vi "Communicator - Passive1.v.vi"() -> ()   [LabVIEW 2019]
panel:
  out "MC_Receive":T1 {"MirrorCoverControlScheme"."Time" format="%<%Y-%m-%d %H:%M:%S>T"; "MirrorCoverControllerConfig"."Time" format="%<%Y-%m-%d %H:%M:%S>T"; "MirrorCoverMotor-All"."MirrorCoverMotor-00"."Time" format="%<%Y-%m-%d %H:%M:%S>T"; "MirrorCoverMotor-All"."MirrorCoverMotor-01"."Time" format="%<%Y-%m-%d %H:%M:%S>T"; "MirrorCoverMotor-All"."MirrorCoverMotor-02"."Time" format="%<%Y-%m-%d %H:%M:%S>T"; "MirrorCoverMotor-All"."MirrorCoverMotor-03"."Time" format="%<%Y-%m-%d %H:%M:%S>T"; "MirrorCoverMotor-All"."MirrorCoverMotor-04"."Time" format="%<%Y-%m-%d %H:%M:%S>T"; "MirrorCoverMotor-All"."MirrorCoverMotor-05"."Time" format="%<%Y-%m-%d %H:%M:%S>T"; "MirrorCoverMotor-All"."MirrorCoverMotor-06"."Time" format="%<%Y-%m-%d %H:%M:%S>T"; "MirrorCoverMotor-All"."MirrorCoverMotor-07"."Time" format="%<%Y-%m-%d %H:%M:%S>T"}
  out "MC_Send 2":T1 {"MirrorCoverControlScheme"."Time" format="%<%Y-%m-%d %H:%M:%S>T"; "MirrorCoverControllerConfig"."Time" format="%<%Y-%m-%d %H:%M:%S>T"; "MirrorCoverMotor-All"."MirrorCoverMotor-00"."Time" format="%<%Y-%m-%d %H:%M:%S>T"; "MirrorCoverMotor-All"."MirrorCoverMotor-01"."Time" format="%<%Y-%m-%d %H:%M:%S>T"; "MirrorCoverMotor-All"."MirrorCoverMotor-02"."Time" format="%<%Y-%m-%d %H:%M:%S>T"; "MirrorCoverMotor-All"."MirrorCoverMotor-03"."Time" format="%<%Y-%m-%d %H:%M:%S>T"; "MirrorCoverMotor-All"."MirrorCoverMotor-04"."Time" format="%<%Y-%m-%d %H:%M:%S>T"; "MirrorCoverMotor-All"."MirrorCoverMotor-05"."Time" format="%<%Y-%m-%d %H:%M:%S>T"; "MirrorCoverMotor-All"."MirrorCoverMotor-06"."Time" format="%<%Y-%m-%d %H:%M:%S>T"; "MirrorCoverMotor-All"."MirrorCoverMotor-07"."Time" format="%<%Y-%m-%d %H:%M:%S>T"}
  in  "MC_Send":T1 {"MirrorCoverControlScheme"."Time" format="%<%Y-%m-%d %H:%M:%S>T"; "MirrorCoverControllerConfig"."Time" format="%<%Y-%m-%d %H:%M:%S>T"; "MirrorCoverMotor-All"."MirrorCoverMotor-00"."Time" format="%<%Y-%m-%d %H:%M:%S>T"; "MirrorCoverMotor-All"."MirrorCoverMotor-01"."Time" format="%<%Y-%m-%d %H:%M:%S>T"; "MirrorCoverMotor-All"."MirrorCoverMotor-02"."Time" format="%<%Y-%m-%d %H:%M:%S>T"; "MirrorCoverMotor-All"."MirrorCoverMotor-03"."Time" format="%<%Y-%m-%d %H:%M:%S>T"; "MirrorCoverMotor-All"."MirrorCoverMotor-04"."Time" format="%<%Y-%m-%d %H:%M:%S>T"; "MirrorCoverMotor-All"."MirrorCoverMotor-05"."Time" format="%<%Y-%m-%d %H:%M:%S>T"; "MirrorCoverMotor-All"."MirrorCoverMotor-06"."Time" format="%<%Y-%m-%d %H:%M:%S>T"; "MirrorCoverMotor-All"."MirrorCoverMotor-07"."Time" format="%<%Y-%m-%d %H:%M:%S>T"}
  in  "Port":u16=6342
  in  "stop":bool
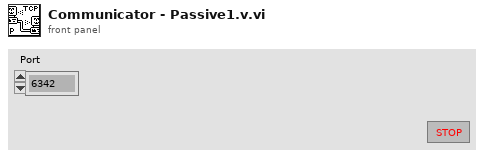
[diagram p1: front panel]
types:
  T1 = cluster{"MirrorCoverControlScheme":cluster{"Cold Start":bool, "Configuration":bool, "Start":bool, "Pointing/Tracking":bool, "Standby":bool, "Stop":bool, "Shutdown":bool, "Start Calibration":bool, "Start Maintenance":bool, "Status":i16, "Time ":timestamp}, "MirrorCoverControllerConfig":cluster{"ID":dbl, "K_P Config":dbl, "K_I Config":dbl, "K_D Config":dbl, "Status":i16, "Time ":timestamp}, "MirrorCoverMotor-All":cluster{"MirrorCoverMotor-00":cluster{"ID":i32, "Enable":bool, "Direction":bool, "Brake":bool, "Built-In Encoder":u64, "Motor Voltage FB":bool, "Motor Current FB":u64, "Brake Voltage FB":bool, "Brake Current FB":u64, "Up Limit Switch":bool, "Down Limit Switch":bool, "Up Limit Config":u64, "Down Limit Config":u64, "Motor Current Limit Config":u64, "Brake Current Limit Config":u64, "Status":i16, "Time ":timestamp}, "MirrorCoverMotor-01":cluster{"ID":i32, "Enable":bool, "Direction":bool, "Brake":bool, "Built-In Encoder":u64, "Motor Voltage FB":bool, "Motor Current FB":u64, "Brake Voltage FB":bool, "Brake Current FB":u64, "Up Limit Switch":bool, "Down Limit Switch":bool, "Up Limit Config":u64, "Down Limit Config":u64, "Motor Current Limit Config":u64, "Brake Current Limit Config":u64, "Status":i16, "Time ":timestamp}, "MirrorCoverMotor-02":cluster{"ID":i32, "Enable":bool, "Direction":bool, "Brake":bool, "Built-In Encoder":u64, "Motor Voltage FB":bool, "Motor Current FB":u64, "Brake Voltage FB":bool, "Brake Current FB":u64, "Up Limit Switch":bool, "Down Limit Switch":bool, "Up Limit Config":u64, "Down Limit Config":u64, "Motor Current Limit Config":u64, "Brake Current Limit Config":u64, "Status":i16, "Time ":timestamp}, "MirrorCoverMotor-03":cluster{"ID":i32, "Enable":bool, "Direction":bool, "Brake":bool, "Built-In Encoder":u64, "Motor Voltage FB":bool, "Motor Current FB":u64, "Brake Voltage FB":bool, "Brake Current FB":u64, "Up Limit Switch":bool, "Down Limit Switch":bool, "Up Limit Config":u64, "Down Limit Config":u64, "Motor Current Limit Config":u64, "Brake Current Limit Config":u64, "Status":i16, "Time ":timestamp}, "MirrorCoverMotor-04":cluster{"ID":i32, "Enable":bool, "Direction":bool, "Brake":bool, "Built-In Encoder":u64, "Motor Voltage FB":bool, "Motor Current FB":u64, "Brake Voltage FB":bool, "Brake Current FB":u64, "Up Limit Switch":bool, "Down Limit Switch":bool, "Up Limit Config":u64, "Down Limit Config":u64, "Motor Current Limit Config":u64, "Brake Current Limit Config":u64, "Status":i16, "Time ":timestamp}, "MirrorCoverMotor-05":cluster{"ID":i32, "Enable":bool, "Direction":bool, "Brake":bool, "Built-In Encoder":u64, "Motor Voltage FB":bool, "Motor Current FB":u64, "Brake Voltage FB":bool, "Brake Current FB":u64, "Up Limit Switch":bool, "Down Limit Switch":bool, "Up Limit Config":u64, "Down Limit Config":u64, "Motor Current Limit Config":u64, "Brake Current Limit Config":u64, "Status":i16, "Time ":timestamp}, "MirrorCoverMotor-06":cluster{"ID":i32, "Enable":bool, "Direction":bool, "Brake":bool, "Built-In Encoder":u64, "Motor Voltage FB":bool, "Motor Current FB":u64, "Brake Voltage FB":bool, "Brake Current FB":u64, "Up Limit Switch":bool, "Down Limit Switch":bool, "Up Limit Config":u64, "Down Limit Config":u64, "Motor Current Limit Config":u64, "Brake Current Limit Config":u64, "Status":i16, "Time ":timestamp}, "MirrorCoverMotor-07":cluster{"ID":i32, "Enable":bool, "Direction":bool, "Brake":bool, "Built-In Encoder":u64, "Motor Voltage FB":bool, "Motor Current FB":u64, "Brake Voltage FB":bool, "Brake Current FB":u64, "Up Limit Switch":bool, "Down Limit Switch":bool, "Up Limit Config":u64, "Down Limit Config":u64, "Motor Current Limit Config":u64, "Brake Current Limit Config":u64, "Status":i16, "Time ":timestamp}}}
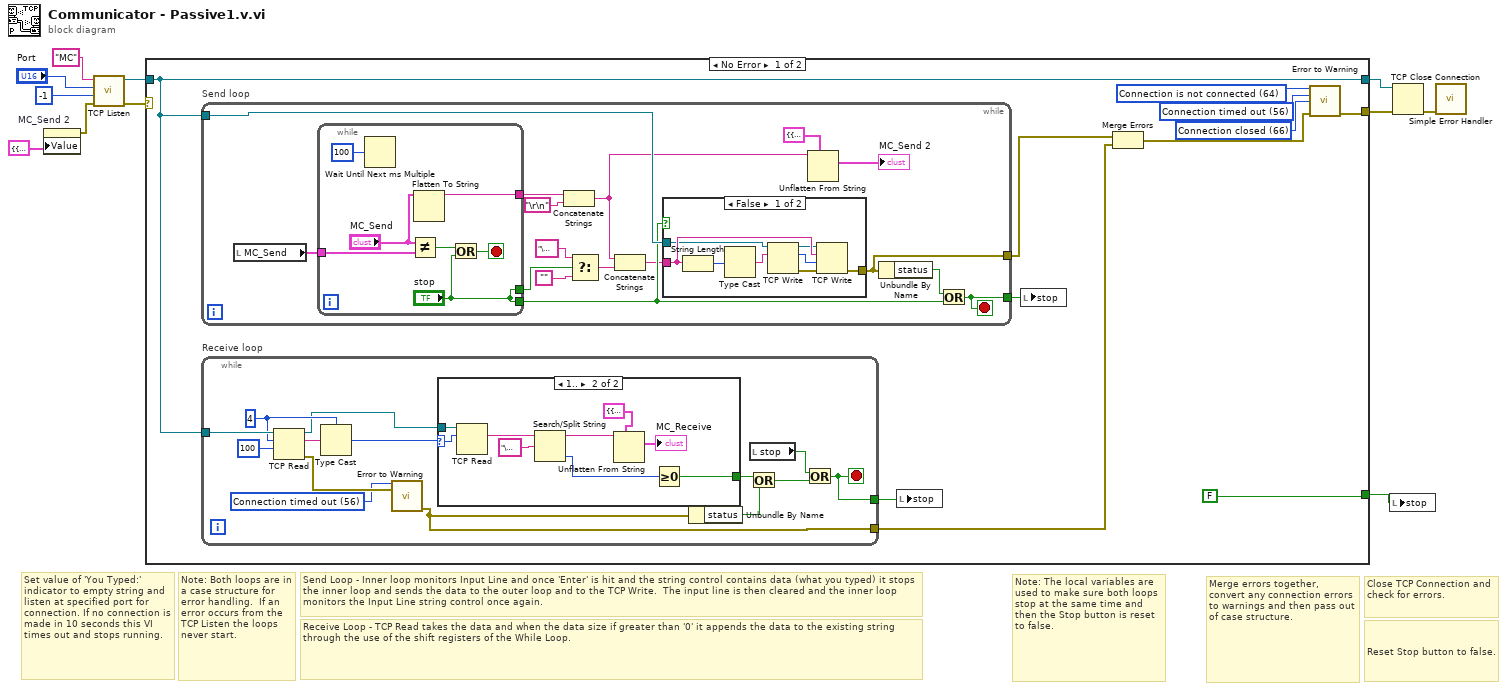
[diagram p0: block diagram]
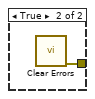
[diagram p2: hidden frame]
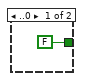
[diagram p3: hidden frame]
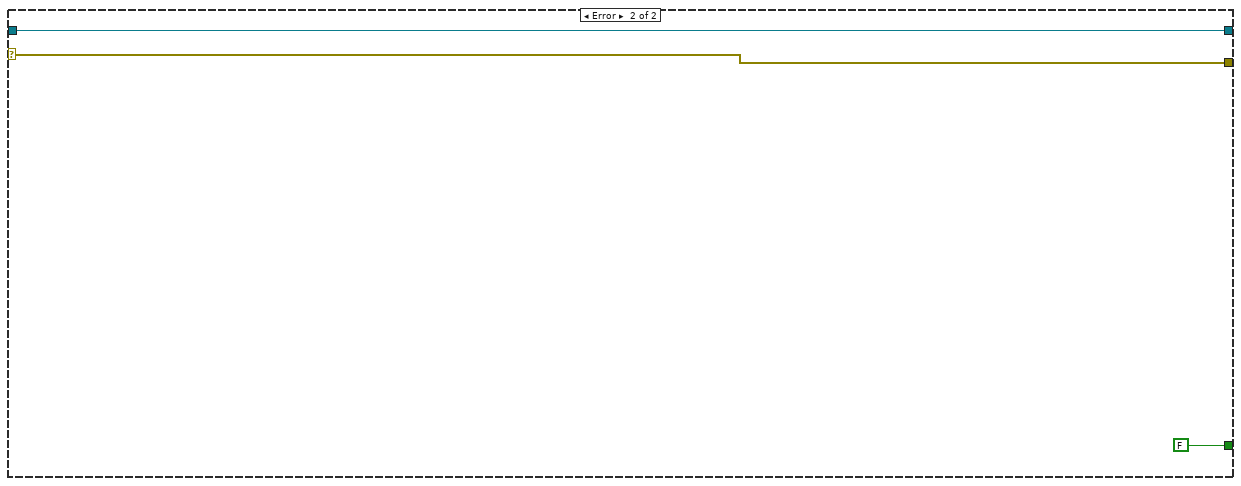
[diagram p4: hidden frame]
diagram:
  # "Reset Stop button to false."
  # "Close TCP Connection and check for errors."
  # "Note: Both loops are in a case structure for error handling.  If an error occurs from the TCP Listen the loops never start."
  # "Merge errors together, convert any connection errors to warnings and then pass out of case structure."
  # "Note: The local variables are used to make sure both loops stop at the same time and then the Stop button is reset to false."
  # "Receive Loop - TCP Read takes the data and when the data size if greater than '0' it appends the data to the existing string through the use of the shift registers of the While Loop."
  # "Send Loop - Inner loop monitors Input Line and once 'Enter' is hit and the string control contains data (what you typed) it stops the inner loop and sends the data to the outer loop and to the TCP Write.  The input line is then cleared and the inner loop monitors the Input Line string control once again."
  # "Set value of 'You Typed:' indicator to empty string and listen at specified port for connection. If no connection is made in 10 seconds this VI times out and stops running."
  n1 = property on="MC_Send 2" class="Clust (strict)"("Value"=T1 {"MirrorCoverControlScheme"={"Cold Start"=FALSE, "Configuration"=FALSE, "Start"=FALSE, "Pointing/Tracking"=FALSE, "Standby"=FALSE, "Stop"=FALSE, "Shutdown"=FALSE, "Start Calibration"=FALSE, "Start Maintenance"=FALSE, "Status"=0, "Time "=timestamp(0 s since 1904-01-01)}, "MirrorCoverControllerConfig"={"ID"=0.0, "K_P Config"=0.0, "K_I Config"=0.0, "K_D Config"=0.0, "Status"=0, "Time "=timestamp(0 s since 1904-01-01)}, "MirrorCoverMotor-All"={"MirrorCoverMotor-00"={"ID"=0, "Enable"=FALSE, "Direction"=FALSE, "Brake"=FALSE, "Built-In Encoder"=0, "Motor Voltage FB"=FALSE, "Motor Current FB"=0, "Brake Voltage FB"=FALSE, "Brake Current FB"=0, "Up Limit Switch"=FALSE, "Down Limit Switch"=FALSE, "Up Limit Config"=0, "Down Limit Config"=0, "Motor Current Limit Config"=0, "Brake Current Limit Config"=0, "Status"=0, "Time "=timestamp(0 s since 1904-01-01)}, "MirrorCoverMotor-01"={"ID"=0, "Enable"=FALSE, "Direction"=FALSE, "Brake"=FALSE, "Built-In Encoder"=0, "Motor Voltage FB"=FALSE, "Motor Current FB"=0, "Brake Voltage FB"=FALSE, "Brake Current FB"=0, "Up Limit Switch"=FALSE, "Down Limit Switch"=FALSE, "Up Limit Config"=0, "Down Limit Config"=0, "Motor Current Limit Config"=0, "Brake Current Limit Config"=0, "Status"=0, "Time "=timestamp(0 s since 1904-01-01)}, "MirrorCoverMotor-02"={"ID"=0, "Enable"=FALSE, "Direction"=FALSE, "Brake"=FALSE, "Built-In Encoder"=0, "Motor Voltage FB"=FALSE, "Motor Current FB"=0, "Brake Voltage FB"=FALSE, "Brake Current FB"=0, "Up Limit Switch"=FALSE, "Down Limit Switch"=FALSE, "Up Limit Config"=0, "Down Limit Config"=0, "Motor Current Limit Config"=0, "Brake Current Limit Config"=0, "Status"=0, "Time "=timestamp(0 s since 1904-01-01)}, "MirrorCoverMotor-03"={"ID"=0, "Enable"=FALSE, "Direction"=FALSE, "Brake"=FALSE, "Built-In Encoder"=0, "Motor Voltage FB"=FALSE, "Motor Current FB"=0, "Brake Voltage FB"=FALSE, "Brake Current FB"=0, "Up Limit Switch"=FALSE, "Down Limit Switch"=FALSE, "Up Limit Config"=0, "Down Limit Config"=0, "Motor Current Limit Config"=0, "Brake Current Limit Config"=0, "Status"=0, "Time "=timestamp(0 s since 1904-01-01)}, "MirrorCoverMotor-04"={"ID"=0, "Enable"=FALSE, "Direction"=FALSE, "Brake"=FALSE, "Built-In Encoder"=0, "Motor Voltage FB"=FALSE, "Motor Current FB"=0, "Brake Voltage FB"=FALSE, "Brake Current FB"=0, "Up Limit Switch"=FALSE, "Down Limit Switch"=FALSE, "Up Limit Config"=0, "Down Limit Config"=0, "Motor Current Limit Config"=0, "Brake Current Limit Config"=0, "Status"=0, "Time "=timestamp(0 s since 1904-01-01)}, "MirrorCoverMotor-05"={"ID"=0, "Enable"=FALSE, "Direction"=FALSE, "Brake"=FALSE, "Built-In Encoder"=0, "Motor Voltage FB"=FALSE, "Motor Current FB"=0, "Brake Voltage FB"=FALSE, "Brake Current FB"=0, "Up Limit Switch"=FALSE, "Down Limit Switch"=FALSE, "Up Limit Config"=0, "Down Limit Config"=0, "Motor Current Limit Config"=0, "Brake Current Limit Config"=0, "Status"=0, "Time "=timestamp(0 s since 1904-01-01)}, "MirrorCoverMotor-06"={"ID"=0, "Enable"=FALSE, "Direction"=FALSE, "Brake"=FALSE, "Built-In Encoder"=0, "Motor Voltage FB"=FALSE, "Motor Current FB"=0, "Brake Voltage FB"=FALSE, "Brake Current FB"=0, "Up Limit Switch"=FALSE, "Down Limit Switch"=FALSE, "Up Limit Config"=0, "Down Limit Config"=0, "Motor Current Limit Config"=0, "Brake Current Limit Config"=0, "Status"=0, "Time "=timestamp(0 s since 1904-01-01)}, "MirrorCoverMotor-07"={"ID"=0, "Enable"=FALSE, "Direction"=FALSE, "Brake"=FALSE, "Built-In Encoder"=0, "Motor Voltage FB"=FALSE, "Motor Current FB"=0, "Brake Voltage FB"=FALSE, "Brake Current FB"=0, "Up Limit Switch"=FALSE, "Down Limit Switch"=FALSE, "Up Limit Config"=0, "Down Limit Config"=0, "Motor Current Limit Config"=0, "Brake Current Limit Config"=0, "Status"=0, "Time "=timestamp(0 s since 1904-01-01)}}} ("MC_Receive")) -> (error out=w6:errorcluster)  [unwired: 2 in, 1 out]
  n2 = call <vilib>:"TCP Listen.vi"("error in (no error)"=w6, "timeout ms (wait forever: -1)"=-1, "port"="Port", "service name"="MC") -> ("error out"=w7:errorcluster, "connection ID"=w8:refnum<k5>)  [unwired: 3 in, 3 out]
  n3 = case shown="No Error" w7 {
    selector: w7 -> [_ w80]
    tunnel: [w17 w80] -> w10
    tunnel: w8 -> [w12 w81]
    tunnel: [w12 w81] -> w11
    tunnel: [FALSE FALSE] -> w3
    frame No Error {
      w14 = 56 items=["No Error", "Argument Error", "Memory Full", "Out of Zone", "End of File", "File Already Open", "Generic File IO Error", "File Not Found", "File Permission Error", "Disk Full", "Duplicate Path", "Too Many Files Open", "Not Enabled", "Resource File Not Found", "Cannot Add Resource", "Resource Not Found", "Image Not Found", "Image Memory Error", "Pen Does Not Exist", "Config Bad Type", "Config Token Not Found", "Config Parse Error", "Config Memory Error", "Bad External Code Format", "Bad External Code Offset", "External Code Not Present", "Null Window", "Destroy Window Mixup", "Null Menu", "Print Aborted", "Bad Print Record", "Print Driver Error", "Windows Error During Print", "Memory Error During Print", "Print Dialog Error", "Generic Print Error", "Invalid Device Refnum", "Device Not Found", "Device Parameter Error", "Device Unit Error", "Can't Open Device", "Device Call Aborted", "Generic Error", "Cancelled By User", "Object ID Too Low", "Object ID Too High", "Object Not In Heap", "Unknown Heap", "Bad DefProc ID", "DefProc Not In Table", "Message Out Of Range", "Null Method", "Unknown Message", "Manager Call Not Supported", "Bad address", "Connection In progress", "Connection timed out", "Connection is already in progress", "Network attribute not supported", "Network error", "Address in use", "System out of memory", "Connection aborted", "Connection refused", "Connection is not connected", "Connection is already connected", "Connection closed", "Initialize error (interapplication manager)", "Bad occurrence", "Wait on unbound occurrence handler", "Occurrence queue overflow", "Bad path", "Semaphore not signaled", "Unrecognized type (interapplication manager)"] ("2nd Error to Convert")
      w18 = 66 items=["No Error", "Argument Error", "Memory Full", "Out of Zone", "End of File", "File Already Open", "Generic File IO Error", "File Not Found", "File Permission Error", "Disk Full", "Duplicate Path", "Too Many Files Open", "Not Enabled", "Resource File Not Found", "Cannot Add Resource", "Resource Not Found", "Image Not Found", "Image Memory Error", "Pen Does Not Exist", "Config Bad Type", "Config Token Not Found", "Config Parse Error", "Config Memory Error", "Bad External Code Format", "Bad External Code Offset", "External Code Not Present", "Null Window", "Destroy Window Mixup", "Null Menu", "Print Aborted", "Bad Print Record", "Print Driver Error", "Windows Error During Print", "Memory Error During Print", "Print Dialog Error", "Generic Print Error", "Invalid Device Refnum", "Device Not Found", "Device Parameter Error", "Device Unit Error", "Can't Open Device", "Device Call Aborted", "Generic Error", "Cancelled By User", "Object ID Too Low", "Object ID Too High", "Object Not In Heap", "Unknown Heap", "Bad DefProc ID", "DefProc Not In Table", "Message Out Of Range", "Null Method", "Unknown Message", "Manager Call Not Supported", "Bad address", "Connection In progress", "Connection timed out", "Connection is already in progress", "Network attribute not supported", "Network error", "Address in use", "System out of memory", "Connection aborted", "Connection refused", "Connection is not connected", "Connection is already connected", "Connection closed", "Initialize error (interapplication manager)", "Bad occurrence", "Wait on unbound occurrence handler", "Occurrence queue overflow", "Bad path", "Semaphore not signaled", "Unrecognized type (interapplication manager)"] ("3rd Error to Convert")
      w19 = 64 items=["No Error", "Argument Error", "Memory Full", "Out of Zone", "End of File", "File Already Open", "Generic File IO Error", "File Not Found", "File Permission Error", "Disk Full", "Duplicate Path", "Too Many Files Open", "Not Enabled", "Resource File Not Found", "Cannot Add Resource", "Resource Not Found", "Image Not Found", "Image Memory Error", "Pen Does Not Exist", "Config Bad Type", "Config Token Not Found", "Config Parse Error", "Config Memory Error", "Bad External Code Format", "Bad External Code Offset", "External Code Not Present", "Null Window", "Destroy Window Mixup", "Null Menu", "Print Aborted", "Bad Print Record", "Print Driver Error", "Windows Error During Print", "Memory Error During Print", "Print Dialog Error", "Generic Print Error", "Invalid Device Refnum", "Device Not Found", "Device Parameter Error", "Device Unit Error", "Can't Open Device", "Device Call Aborted", "Generic Error", "Cancelled By User", "Object ID Too Low", "Object ID Too High", "Object Not In Heap", "Unknown Heap", "Bad DefProc ID", "DefProc Not In Table", "Message Out Of Range", "Null Method", "Unknown Message", "Manager Call Not Supported", "Bad address", "Connection In progress", "Connection timed out", "Connection is already in progress", "Network attribute not supported", "Network error", "Address in use", "System out of memory", "Connection aborted", "Connection refused", "Connection is not connected", "Connection is already connected", "Connection closed", "Initialize error (interapplication manager)", "Bad occurrence", "Wait on unbound occurrence handler", "Occurrence queue overflow", "Bad path", "Semaphore not signaled", "Unrecognized type (interapplication manager)"] ("1st Error to Convert")
      n4 = while "Send loop" {
        tunnel: w12 -> [w37]
        tunnel: [w38] -> w15
        tunnel: [w33] -> w21
        stop <- w38 stop-if-true
        n5 = local read "MC_Send"() -> (w30:T1)
        n6 = while {
          tunnel: ["stop"] -> w35
          tunnel: ["stop"] -> w31
          tunnel: [w39] -> w26
          tunnel: w30 -> [w42]
          stop <- w43 stop-if-true
          n7 = Wait Until Next ms Multiple(millisecond multiple=u32 100) -> ()  [unwired: 1 out]
          n8 = Not Equal?(x="MC_Send", y=w42) -> (x != y?=w44:bool)
          n9 = Flatten To String(anything="MC_Send") -> (data string=w39:string)  [unwired: 3 in, 2 out]
          n10 = Or(x=w44, y="stop") -> (x .or. y?=w43:bool)
        }
        n11 = Concatenate Strings(w26, "\r\n") -> (w25:string)
        n12 = Select(t="\u0004", s=w35, f="") -> (s? t:f=w24:string)
        n13 = Concatenate Strings(w25, w24) -> (w23:string)
        n14 = case shown="False" w31 {
          tunnel: w23 -> [w50 _]
          tunnel: [w53 w54] -> w33
          tunnel: w37 -> [w47 _]
          frame False {
            n15 = String Length(string=w50) -> (length=w49:i32)
            n16 = Type Cast(x=w49) -> (*(type *) &x=w48:string)  [unwired: 1 in]
            n17 = TCP Write(connection ID=w47, data in=w48) -> (connection ID out=w46:refnum<k5>, bytes written=w51:i32, error out=w52:errorcluster)  [unwired: 2 in]
            n18 = TCP Write(connection ID=w46, data in=w50, error in (no error)=w52, 9:w51) -> (error out=w53:errorcluster)  [unwired: 2 out]
          }
          frame True {
            n19 = call <vilib>:"Clear Errors.vi"() -> ("error out"=w54:errorcluster)  [unwired: 6 in, 1 out]
          }
        }
        n20 = Unflatten From String(type=T1 {"MirrorCoverControlScheme"={"Cold Start"=FALSE, "Configuration"=FALSE, "Start"=FALSE, "Pointing/Tracking"=FALSE, "Standby"=FALSE, "Stop"=FALSE, "Shutdown"=FALSE, "Start Calibration"=FALSE, "Start Maintenance"=FALSE, "Status"=0, "Time "=timestamp(0 s since 1904-01-01)}, "MirrorCoverControllerConfig"={"ID"=0.0, "K_P Config"=0.0, "K_I Config"=0.0, "K_D Config"=0.0, "Status"=0, "Time "=timestamp(0 s since 1904-01-01)}, "MirrorCoverMotor-All"={"MirrorCoverMotor-00"={"ID"=0, "Enable"=FALSE, "Direction"=FALSE, "Brake"=FALSE, "Built-In Encoder"=0, "Motor Voltage FB"=FALSE, "Motor Current FB"=0, "Brake Voltage FB"=FALSE, "Brake Current FB"=0, "Up Limit Switch"=FALSE, "Down Limit Switch"=FALSE, "Up Limit Config"=0, "Down Limit Config"=0, "Motor Current Limit Config"=0, "Brake Current Limit Config"=0, "Status"=0, "Time "=timestamp(0 s since 1904-01-01)}, "MirrorCoverMotor-01"={"ID"=0, "Enable"=FALSE, "Direction"=FALSE, "Brake"=FALSE, "Built-In Encoder"=0, "Motor Voltage FB"=FALSE, "Motor Current FB"=0, "Brake Voltage FB"=FALSE, "Brake Current FB"=0, "Up Limit Switch"=FALSE, "Down Limit Switch"=FALSE, "Up Limit Config"=0, "Down Limit Config"=0, "Motor Current Limit Config"=0, "Brake Current Limit Config"=0, "Status"=0, "Time "=timestamp(0 s since 1904-01-01)}, "MirrorCoverMotor-02"={"ID"=0, "Enable"=FALSE, "Direction"=FALSE, "Brake"=FALSE, "Built-In Encoder"=0, "Motor Voltage FB"=FALSE, "Motor Current FB"=0, "Brake Voltage FB"=FALSE, "Brake Current FB"=0, "Up Limit Switch"=FALSE, "Down Limit Switch"=FALSE, "Up Limit Config"=0, "Down Limit Config"=0, "Motor Current Limit Config"=0, "Brake Current Limit Config"=0, "Status"=0, "Time "=timestamp(0 s since 1904-01-01)}, "MirrorCoverMotor-03"={"ID"=0, "Enable"=FALSE, "Direction"=FALSE, "Brake"=FALSE, "Built-In Encoder"=0, "Motor Voltage FB"=FALSE, "Motor Current FB"=0, "Brake Voltage FB"=FALSE, "Brake Current FB"=0, "Up Limit Switch"=FALSE, "Down Limit Switch"=FALSE, "Up Limit Config"=0, "Down Limit Config"=0, "Motor Current Limit Config"=0, "Brake Current Limit Config"=0, "Status"=0, "Time "=timestamp(0 s since 1904-01-01)}, "MirrorCoverMotor-04"={"ID"=0, "Enable"=FALSE, "Direction"=FALSE, "Brake"=FALSE, "Built-In Encoder"=0, "Motor Voltage FB"=FALSE, "Motor Current FB"=0, "Brake Voltage FB"=FALSE, "Brake Current FB"=0, "Up Limit Switch"=FALSE, "Down Limit Switch"=FALSE, "Up Limit Config"=0, "Down Limit Config"=0, "Motor Current Limit Config"=0, "Brake Current Limit Config"=0, "Status"=0, "Time "=timestamp(0 s since 1904-01-01)}, "MirrorCoverMotor-05"={"ID"=0, "Enable"=FALSE, "Direction"=FALSE, "Brake"=FALSE, "Built-In Encoder"=0, "Motor Voltage FB"=FALSE, "Motor Current FB"=0, "Brake Voltage FB"=FALSE, "Brake Current FB"=0, "Up Limit Switch"=FALSE, "Down Limit Switch"=FALSE, "Up Limit Config"=0, "Down Limit Config"=0, "Motor Current Limit Config"=0, "Brake Current Limit Config"=0, "Status"=0, "Time "=timestamp(0 s since 1904-01-01)}, "MirrorCoverMotor-06"={"ID"=0, "Enable"=FALSE, "Direction"=FALSE, "Brake"=FALSE, "Built-In Encoder"=0, "Motor Voltage FB"=FALSE, "Motor Current FB"=0, "Brake Voltage FB"=FALSE, "Brake Current FB"=0, "Up Limit Switch"=FALSE, "Down Limit Switch"=FALSE, "Up Limit Config"=0, "Down Limit Config"=0, "Motor Current Limit Config"=0, "Brake Current Limit Config"=0, "Status"=0, "Time "=timestamp(0 s since 1904-01-01)}, "MirrorCoverMotor-07"={"ID"=0, "Enable"=FALSE, "Direction"=FALSE, "Brake"=FALSE, "Built-In Encoder"=0, "Motor Voltage FB"=FALSE, "Motor Current FB"=0, "Brake Voltage FB"=FALSE, "Brake Current FB"=0, "Up Limit Switch"=FALSE, "Down Limit Switch"=FALSE, "Up Limit Config"=0, "Down Limit Config"=0, "Motor Current Limit Config"=0, "Brake Current Limit Config"=0, "Status"=0, "Time "=timestamp(0 s since 1904-01-01)}}} ("MC_Receive"), binary string=w25) -> (value=→"MC_Send 2":T1)  [unwired: 3 in, 2 out]
        n21 = Unbundle By Name(w33) -> ("status"=w32:bool)
        n22 = Or(x=w32, y=w31) -> (x .or. y?=w38:bool)
      }
      n23 = while "Receive loop" {
        tunnel: [w67] -> w16
        tunnel: [w62] -> w22
        tunnel: w12 -> [w68]
        stop <- w67 stop-if-true
        w57 = 4
        w63 = 56 items=["No Error", "Argument Error", "Memory Full", "Out of Zone", "End of File", "File Already Open", "Generic File IO Error", "File Not Found", "File Permission Error", "Disk Full", "Duplicate Path", "Too Many Files Open", "Not Enabled", "Resource File Not Found", "Cannot Add Resource", "Resource Not Found", "Image Not Found", "Image Memory Error", "Pen Does Not Exist", "Config Bad Type", "Config Token Not Found", "Config Parse Error", "Config Memory Error", "Bad External Code Format", "Bad External Code Offset", "External Code Not Present", "Null Window", "Destroy Window Mixup", "Null Menu", "Print Aborted", "Bad Print Record", "Print Driver Error", "Windows Error During Print", "Memory Error During Print", "Print Dialog Error", "Generic Print Error", "Invalid Device Refnum", "Device Not Found", "Device Parameter Error", "Device Unit Error", "Can't Open Device", "Device Call Aborted", "Generic Error", "Cancelled By User", "Object ID Too Low", "Object ID Too High", "Object Not In Heap", "Unknown Heap", "Bad DefProc ID", "DefProc Not In Table", "Message Out Of Range", "Null Method", "Unknown Message", "Manager Call Not Supported", "Bad address", "Connection In progress", "Connection timed out", "Connection is already in progress", "Network attribute not supported", "Network error", "Address in use", "System out of memory", "Connection aborted", "Connection refused", "Connection is not connected", "Connection is already connected", "Connection closed", "Initialize error (interapplication manager)", "Bad occurrence", "Wait on unbound occurrence handler", "Occurrence queue overflow", "Bad path", "Semaphore not signaled", "Unrecognized type (interapplication manager)"] ("1st Error to Convert")
        n24 = TCP Read(connection ID=w68, bytes to read=w57, 9:100) -> (connection ID out=w55:refnum<k5>, data out=w58:string, error out=w64:errorcluster)  [unwired: 2 in]
        n25 = Type Cast(type=w57, x=w58) -> (*(type *) &x=w56:i32)
        n26 = call <vilib>:"Error to Warning.vi"("1st Error to Convert"=w63, "error in"=w64) -> ("warning out"=w62:errorcluster)  [unwired: 13 in]
        n27 = case shown="1.." w56 {
          selector: w56 -> [_ w78]
          tunnel: [FALSE w73] -> w66
          tunnel: w55 -> [_ w77]
          frame ..0 {
          }
          frame 1.. {
            n28 = TCP Read(connection ID=w77, bytes to read=w78) -> (data out=w72:string)  [unwired: 3 in, 2 out]
            n29 = Search/Split String(string=w72, search string/char (-)="\u0004") -> (substring before match=w71:string, offset of match=w75:i32)  [unwired: 1 in, 1 out]
            n30 = Unflatten From String(type=T1 {"MirrorCoverControlScheme"={"Cold Start"=FALSE, "Configuration"=FALSE, "Start"=FALSE, "Pointing/Tracking"=FALSE, "Standby"=FALSE, "Stop"=FALSE, "Shutdown"=FALSE, "Start Calibration"=FALSE, "Start Maintenance"=FALSE, "Status"=0, "Time "=timestamp(0 s since 1904-01-01)}, "MirrorCoverControllerConfig"={"ID"=0.0, "K_P Config"=0.0, "K_I Config"=0.0, "K_D Config"=0.0, "Status"=0, "Time "=timestamp(0 s since 1904-01-01)}, "MirrorCoverMotor-All"={"MirrorCoverMotor-00"={"ID"=0, "Enable"=FALSE, "Direction"=FALSE, "Brake"=FALSE, "Built-In Encoder"=0, "Motor Voltage FB"=FALSE, "Motor Current FB"=0, "Brake Voltage FB"=FALSE, "Brake Current FB"=0, "Up Limit Switch"=FALSE, "Down Limit Switch"=FALSE, "Up Limit Config"=0, "Down Limit Config"=0, "Motor Current Limit Config"=0, "Brake Current Limit Config"=0, "Status"=0, "Time "=timestamp(0 s since 1904-01-01)}, "MirrorCoverMotor-01"={"ID"=0, "Enable"=FALSE, "Direction"=FALSE, "Brake"=FALSE, "Built-In Encoder"=0, "Motor Voltage FB"=FALSE, "Motor Current FB"=0, "Brake Voltage FB"=FALSE, "Brake Current FB"=0, "Up Limit Switch"=FALSE, "Down Limit Switch"=FALSE, "Up Limit Config"=0, "Down Limit Config"=0, "Motor Current Limit Config"=0, "Brake Current Limit Config"=0, "Status"=0, "Time "=timestamp(0 s since 1904-01-01)}, "MirrorCoverMotor-02"={"ID"=0, "Enable"=FALSE, "Direction"=FALSE, "Brake"=FALSE, "Built-In Encoder"=0, "Motor Voltage FB"=FALSE, "Motor Current FB"=0, "Brake Voltage FB"=FALSE, "Brake Current FB"=0, "Up Limit Switch"=FALSE, "Down Limit Switch"=FALSE, "Up Limit Config"=0, "Down Limit Config"=0, "Motor Current Limit Config"=0, "Brake Current Limit Config"=0, "Status"=0, "Time "=timestamp(0 s since 1904-01-01)}, "MirrorCoverMotor-03"={"ID"=0, "Enable"=FALSE, "Direction"=FALSE, "Brake"=FALSE, "Built-In Encoder"=0, "Motor Voltage FB"=FALSE, "Motor Current FB"=0, "Brake Voltage FB"=FALSE, "Brake Current FB"=0, "Up Limit Switch"=FALSE, "Down Limit Switch"=FALSE, "Up Limit Config"=0, "Down Limit Config"=0, "Motor Current Limit Config"=0, "Brake Current Limit Config"=0, "Status"=0, "Time "=timestamp(0 s since 1904-01-01)}, "MirrorCoverMotor-04"={"ID"=0, "Enable"=FALSE, "Direction"=FALSE, "Brake"=FALSE, "Built-In Encoder"=0, "Motor Voltage FB"=FALSE, "Motor Current FB"=0, "Brake Voltage FB"=FALSE, "Brake Current FB"=0, "Up Limit Switch"=FALSE, "Down Limit Switch"=FALSE, "Up Limit Config"=0, "Down Limit Config"=0, "Motor Current Limit Config"=0, "Brake Current Limit Config"=0, "Status"=0, "Time "=timestamp(0 s since 1904-01-01)}, "MirrorCoverMotor-05"={"ID"=0, "Enable"=FALSE, "Direction"=FALSE, "Brake"=FALSE, "Built-In Encoder"=0, "Motor Voltage FB"=FALSE, "Motor Current FB"=0, "Brake Voltage FB"=FALSE, "Brake Current FB"=0, "Up Limit Switch"=FALSE, "Down Limit Switch"=FALSE, "Up Limit Config"=0, "Down Limit Config"=0, "Motor Current Limit Config"=0, "Brake Current Limit Config"=0, "Status"=0, "Time "=timestamp(0 s since 1904-01-01)}, "MirrorCoverMotor-06"={"ID"=0, "Enable"=FALSE, "Direction"=FALSE, "Brake"=FALSE, "Built-In Encoder"=0, "Motor Voltage FB"=FALSE, "Motor Current FB"=0, "Brake Voltage FB"=FALSE, "Brake Current FB"=0, "Up Limit Switch"=FALSE, "Down Limit Switch"=FALSE, "Up Limit Config"=0, "Down Limit Config"=0, "Motor Current Limit Config"=0, "Brake Current Limit Config"=0, "Status"=0, "Time "=timestamp(0 s since 1904-01-01)}, "MirrorCoverMotor-07"={"ID"=0, "Enable"=FALSE, "Direction"=FALSE, "Brake"=FALSE, "Built-In Encoder"=0, "Motor Voltage FB"=FALSE, "Motor Current FB"=0, "Brake Voltage FB"=FALSE, "Brake Current FB"=0, "Up Limit Switch"=FALSE, "Down Limit Switch"=FALSE, "Up Limit Config"=0, "Down Limit Config"=0, "Motor Current Limit Config"=0, "Brake Current Limit Config"=0, "Status"=0, "Time "=timestamp(0 s since 1904-01-01)}}} ("MC_Receive"), binary string=w71) -> (value=→"MC_Receive":T1)  [unwired: 3 in, 2 out]
            n31 = Greater Or Equal To 0?(x=w75) -> (x >= 0?=w73:bool)
          }
        }
        n32 = Unbundle By Name(w62) -> ("status"=w61:bool)
        n33 = Or(x=w66, y=w61) -> (x .or. y?=w59:bool)
        n34 = local read "stop"() -> (w60:bool)
        n35 = Or(x=w60, y=w59) -> (x .or. y?=w67:bool)
      }
      n36 = local write "stop"(w16) -> ()
      n37 = local write "stop"(w15) -> ()
      n38 = Merge Errors(w21, w22) -> (w20:errorcluster)
      n39 = call <vilib>:"Error to Warning.vi"("1st Error to Convert"=w19, "2nd Error to Convert"=w14, "3rd Error to Convert"=w18, "error in"=w20) -> ("warning out"=w17:errorcluster)  [unwired: 11 in]
    }
    frame Error {
    }
  }
  n40 = local write "stop"(w3) -> ()
  n41 = TCP Close Connection(connection ID=w11, error in (no error)=w10) -> (error out=w9:errorcluster)  [unwired: 1 in, 1 out]
  n42 = call <vilib>:"Simple Error Handler.vi"("error in (no error)"=w9) -> ()  [unwired: 4 in, 5 out]
